vi "test2.vi"() -> ()   [LabVIEW 2014]
panel:
  in  "Cluster":T1
  in  "stop":bool
  out "String":string="pressed"
  out "Char":i16
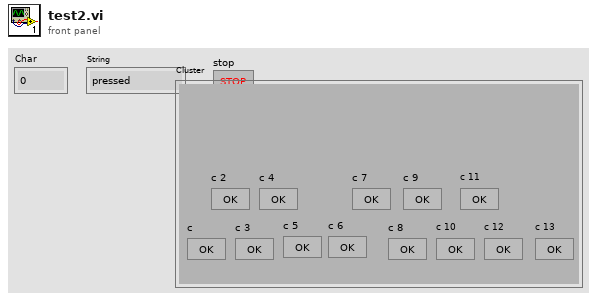
[diagram p1: front panel]
types:
  T1 = cluster{"c":bool, "c 2":bool, "c 3":bool, "c 4":bool, "c 5":bool, "c 6":bool, "c 7":bool, "c 8":bool, "c 9":bool, "c 10":bool, "c 11":bool, "c 12":bool, "c 13":bool}
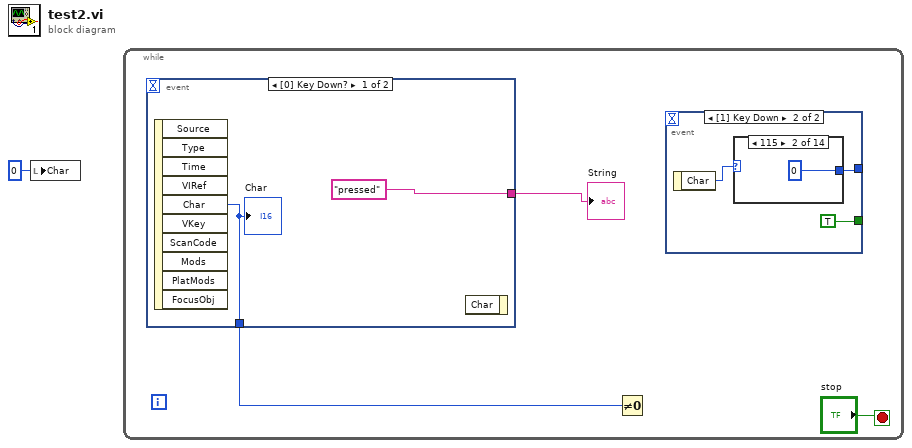
[diagram p0: block diagram]
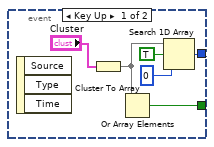
[diagram p2: hidden frame]
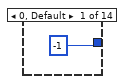
[diagram p3: hidden frame]
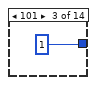
[diagram p4: hidden frame]
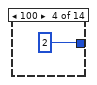
[diagram p5: hidden frame]
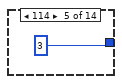
[diagram p6: hidden frame]
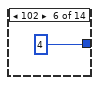
[diagram p7: hidden frame]
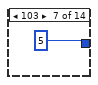
[diagram p8: hidden frame]
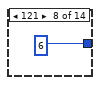
[diagram p9: hidden frame]
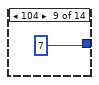
[diagram p10: hidden frame]
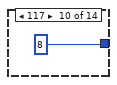
[diagram p11: hidden frame]
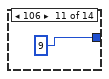
[diagram p12: hidden frame]
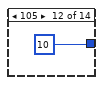
[diagram p13: hidden frame]
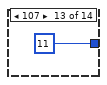
[diagram p14: hidden frame]
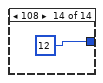
[diagram p15: hidden frame]
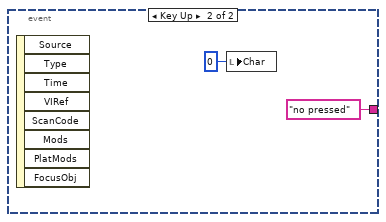
[diagram p16: hidden frame]
diagram:
  n1 = local write "Char"(i16 0 ("Char")) -> ()
  n2 = while {
    stop <- "stop" stop-if-true
    n3 = event shown="[0] Key Down?" {
      selector: _ -> [_ _]
      dyn-events: _ -> [_ _]
      timeout: _ -> [_ _]
      tunnel: [w29 _] -> w4
      tunnel: ["pressed" "no pressed"] -> w3
      event Key Down? {
        n4 = event-data() -> ("Char"=w29:i16)  [unwired: 1 in, 9 out]
        "Char" <- w29
        n5 = event-data() -> ()  [unwired: 2 in, 1 out]
      }
      event Key Up {
        n6 = event-data() -> ()  [unwired: 1 in, 8 out]
        n7 = local write "Char"(i16 0 ("Char")) -> ()
      }
    }
    "String" <- w3
    n8 = Not Equal To 0?(x=w4) -> ()  [unwired: 1 out]
    n9 = event shown="[1] Key Down" {
      selector: _ -> [_ _]
      dyn-events: _ -> [_ _]
      timeout: _ -> [_ _]
      tunnel: [w9 TRUE] -> _
      tunnel: [w5 w12] -> _
      event Key Up {
        n10 = event-data() -> ()  [unwired: 1 in, 3 out]
        n11 = Cluster To Array(cluster="Cluster") -> (array=w8:bool[])
        n12 = Or Array Elements(Boolean array=w8) -> (logical OR=w9:bool)
        n13 = Search 1D Array(1D array=w8, element=TRUE, start index (0)=0) -> (index of element=w5:i32)
      }
      event Key Down {
        n14 = event-data() -> ("Char"=w13:i16)  [unwired: 1 in]
        n15 = case shown="115" w13 {
          tunnel: [-1 0 1 2 3 4 5 6 7 8 9 10 11 12] -> w12
          frame 0, Default {
          }
          frame 115 {
          }
          frame 101 {
          }
          frame 100 {
          }
          frame 114 {
          }
          frame 102 {
          }
          frame 103 {
          }
          frame 121 {
          }
          frame 104 {
          }
          frame 117 {
          }
          frame 106 {
          }
          frame 105 {
          }
          frame 107 {
          }
          frame 108 {
          }
        }
      }
    }
  }
